vi "Parse-broadcast-data-status.vi"(8 "error in (no error)":errorcluster, 10 "Multiple device identification XML string":string="<LecList>\n  <Lec name='EC_Alpha' ip='192.168.42.30' mac='address' />\n  <Lec name='EC_Beta' ip='192.168.42.31' mac='addressB' />\n</LecList>") -> (0 "error out":errorcluster, 2 "Status information":T1)   [LabVIEW 2013, in "HardwareCharacterization.lvlib" / "HC-SM1000.lvclass"]
uses:
  HC-SM1000.lvclass
  Status-information.ctl
  <vilib>/xml/Load XML String.vi
  <vilib>/xml/Close Reference(Node).vi
  <vilib>/xml/NI_XML.lvlib
  <resource>/objmgr/DOMUserDefRef.rc
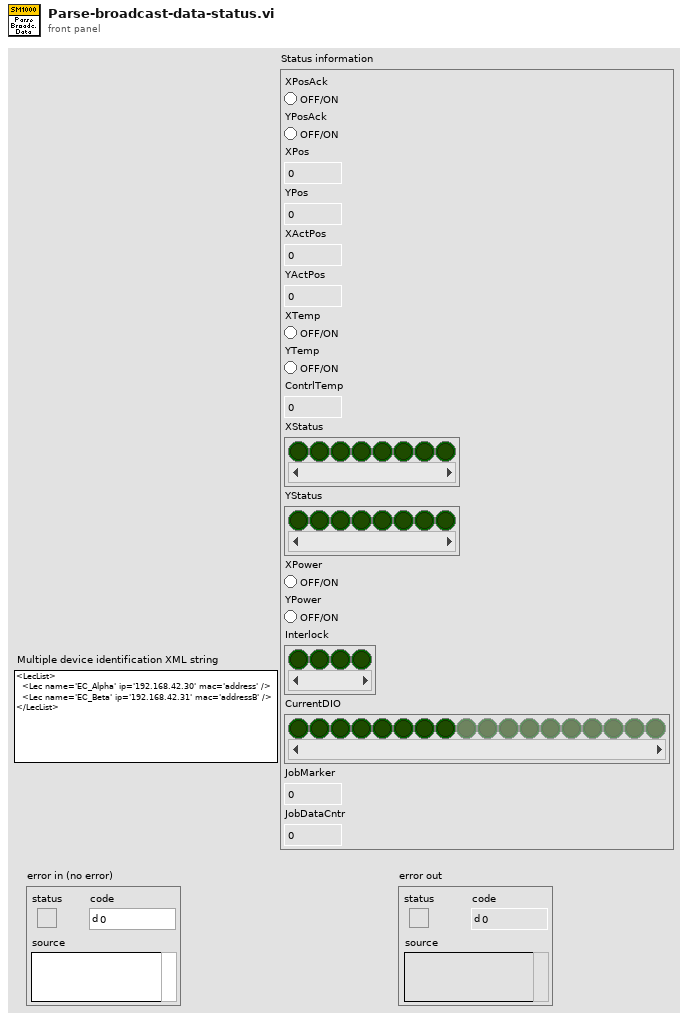
[diagram p1: front panel]
types:
  T1 = typedef "HardwareCharacterization.lvlib/HC-SM1000.lvclass/Status-information.ctl" = cluster{"XPosAck":bool, "YPosAck":bool, "XPos":i16, "YPos":i16, "XActPos":i16, "YActPos":i16, "XTemp":bool, "YTemp":bool, "ContrlTemp":i16, "XStatus":bool[], "YStatus":bool[], "XPower":bool, "YPower":bool, "Interlock":bool[], "CurrentDIO":bool[], "JobMarker":u16, "JobDataCntr":u32}
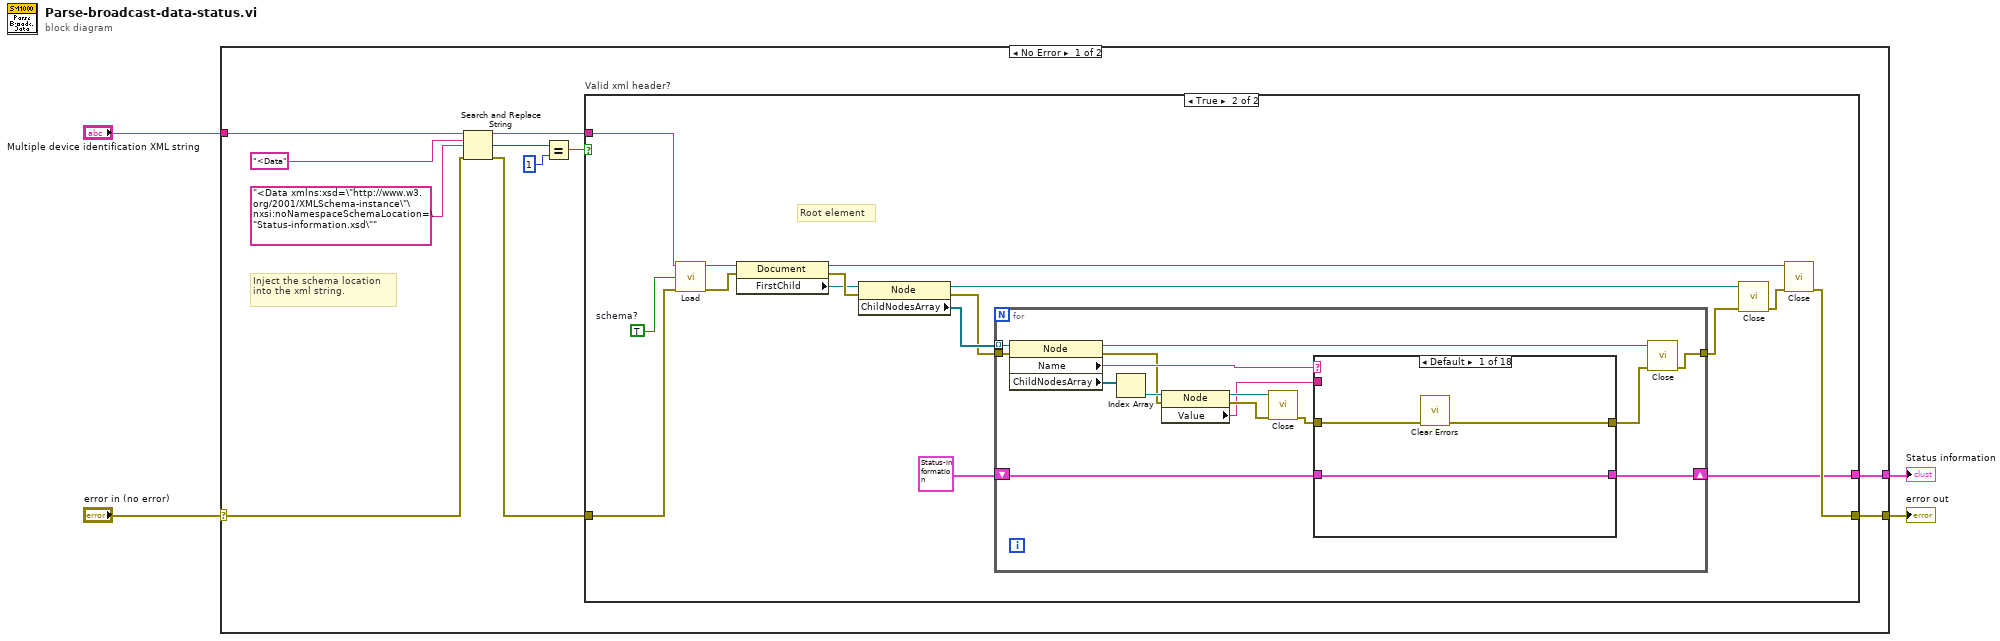
[diagram p0: block diagram]
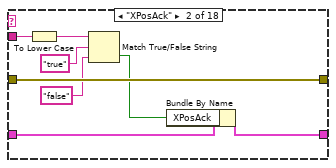
[diagram p3: hidden frame]
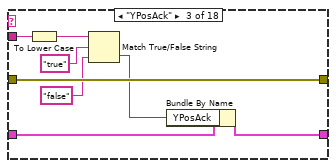
[diagram p4: hidden frame]
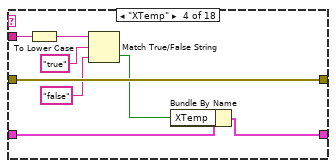
[diagram p5: hidden frame]
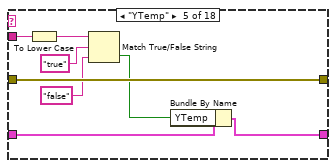
[diagram p6: hidden frame]
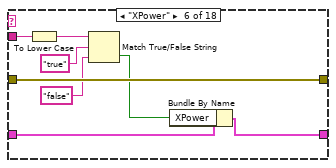
[diagram p7: hidden frame]
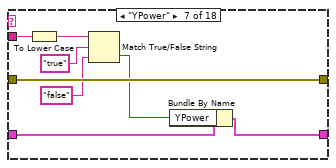
[diagram p8: hidden frame]
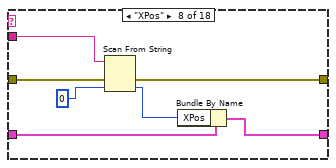
[diagram p9: hidden frame]
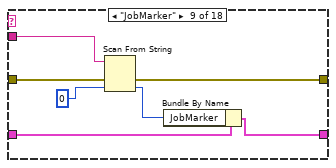
[diagram p10: hidden frame]
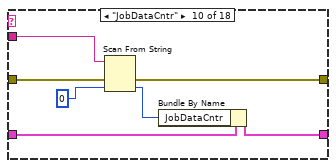
[diagram p11: hidden frame]
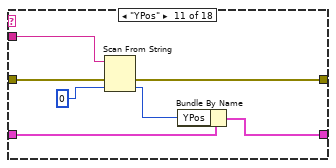
[diagram p12: hidden frame]
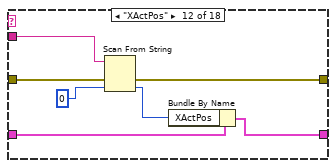
[diagram p13: hidden frame]
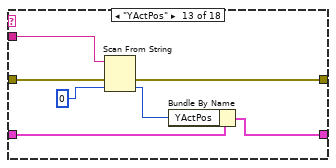
[diagram p14: hidden frame]
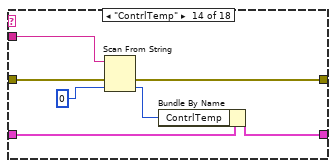
[diagram p15: hidden frame]
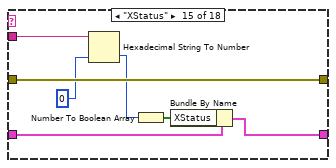
[diagram p16: hidden frame]
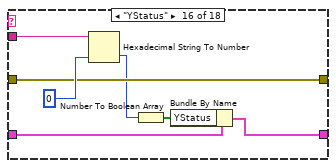
[diagram p17: hidden frame]
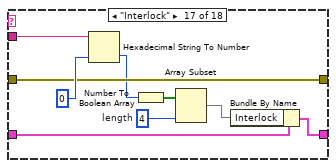
[diagram p18: hidden frame]
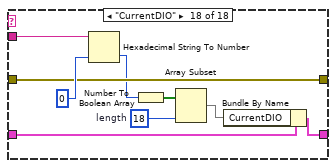
[diagram p19: hidden frame]
diagram:
  n1 = case shown="No Error" "error in (no error)" {
    selector: "error in (no error)" -> [w12 w180]
    tunnel: [w7 w180] -> w3
    tunnel: "Multiple device identification XML string" -> [w15 _]
    tunnel: [w5 _] -> w1
    frame No Error {
      # "Inject the schema location\ninto the xml string."
      n2 = Search and Replace String(input string=w15, search string="<Data", replace string="<Data xmlns:xsd=\"http://www.w3.org/2001/XMLSchema-instance\"\nxsi:noNamespaceSchemaLocation=\"Status-information.xsd\"", error in=w12) -> (result string=w8:string, number of replacements=w11:i32, error out=w6:errorcluster)  [unwired: 4 in, 1 out]
      n3 = Equal?(x=w11, y=1) -> (x = y?=w9:bool)
      n4 = case "Valid xml header?" shown="True" w9 {
        tunnel: w8 -> [_ w19]
        tunnel: [w16 w28] -> w7
        tunnel: w6 -> [w16 w29]
        tunnel: [_ w17] -> w5
        frame False {
        }
        frame True {
          w32 = TRUE  # schema?
          # "Root element"
          n5 = call-poly <vilib>:"Load.vi"("XML string"=w19, "process schema (False)"=w32, "error in (no error)"=w29) -> ("DOM document out"=w31:refnum<k20>, "error out"=w30:errorcluster)  [unwired: 10 in, 1 out]
          n6 = property class="Document"(reference=w31, error in=w30) -> (reference out=w21:refnum<k20>, error out=w23:errorcluster, "FirstChild"=w20:refnum<k20>)
          n7 = property class="Node"(reference=w20, error in=w23) -> (reference out=w22:refnum<k20>, error out=w24:errorcluster, "ChildNodesArray"=w25:refnum<k20>[])
          n8 = for {
            tunnel: w25 -> [w47] mode=indexing
            tunnel: w24 -> [w46]
            tunnel: [w43] -> w27
            shift-right: [w40] -> w17
            shift-left: T1 {"XPosAck"=FALSE, "YPosAck"=FALSE, "XPos"=0, "YPos"=0, "XActPos"=0, "YActPos"=0, "XTemp"=FALSE, "YTemp"=FALSE, "ContrlTemp"=0, "XStatus"=[FALSE, FALSE, FALSE, FALSE, FALSE, FALSE, FALSE, FALSE], "YStatus"=[FALSE, FALSE, FALSE, FALSE, FALSE, FALSE, FALSE, FALSE], "XPower"=FALSE, "YPower"=FALSE, "Interlock"=[FALSE, FALSE, FALSE, FALSE], "CurrentDIO"=[FALSE, FALSE, FALSE, FALSE, FALSE, FALSE, FALSE, FALSE, FALSE, FALSE, FALSE, FALSE, FALSE, FALSE, FALSE, FALSE, FALSE, FALSE], "JobMarker"=0, "JobDataCntr"=0} ("Status information") -> [w41]
            n9 = property class="Node"(reference=w47, error in=w46) -> (reference out=w45:refnum<k20>, error out=w37:errorcluster, "Name"=w42:string, "ChildNodesArray"=w39:refnum<k20>[])
            n10 = Index Array(array=w39) -> (element=w38:refnum<k20>)  [unwired: 1 in]
            n11 = property class="Node"(reference=w38, error in=w37) -> (reference out=w34:refnum<k20>, error out=w36:errorcluster, "Value"=w33:string)
            n12 = call-poly <vilib>:"Close.vi"("error in (no error)"=w36, "node"=w34) -> ("error out"=w35:errorcluster)  [unwired: 7 in]
            n13 = case shown="Default" w42 {
              tunnel: w35 -> [w50 w55 w63 w71 w79 w87 w95 w103 w110 w117 w124 w131 w138 w145 w150 w156 w163 w172]
              tunnel: [w48 w55 w63 w71 w79 w87 w95 w99 w106 w113 w120 w127 w134 w141 w150 w156 w163 w172] -> w44
              tunnel: w41 -> [w49 w58 w66 w74 w82 w90 w98 w105 w112 w119 w126 w133 w140 w147 w154 w161 w170 w179]
              tunnel: w33 -> [_ w56 w64 w72 w80 w88 w96 w102 w109 w116 w123 w130 w137 w144 w152 w157 w164 w173]
              tunnel: [w49 w57 w65 w73 w81 w89 w97 w104 w111 w118 w125 w132 w139 w146 w153 w160 w169 w178] -> w40
              frame Default {
                n14 = call <vilib>:"Clear Errors.vi"("error in (no error)"=w50) -> ("error out"=w48:errorcluster)  [unwired: 6 in]
              }
              frame "XPosAck" {
                n15 = To Lower Case(string=w56) -> (all lower case string=w54:string)
                n16 = Match True/False String(2:"false", 3:"true", 4:w54) -> (0:w51:bool)  [unwired: 1 out]
                n17 = Bundle By Name(cluster=w58, "XPosAck"=w51) -> (w57:T1)
              }
              frame "YPosAck" {
                n18 = To Lower Case(string=w64) -> (all lower case string=w62:string)
                n19 = Match True/False String(2:"false", 3:"true", 4:w62) -> (0:w59:bool)  [unwired: 1 out]
                n20 = Bundle By Name(cluster=w66, "YPosAck"=w59) -> (w65:T1)
              }
              frame "XTemp" {
                n21 = To Lower Case(string=w72) -> (all lower case string=w70:string)
                n22 = Match True/False String(2:"false", 3:"true", 4:w70) -> (0:w67:bool)  [unwired: 1 out]
                n23 = Bundle By Name(cluster=w74, "XTemp"=w67) -> (w73:T1)
              }
              frame "YTemp" {
                n24 = To Lower Case(string=w80) -> (all lower case string=w78:string)
                n25 = Match True/False String(2:"false", 3:"true", 4:w78) -> (0:w75:bool)  [unwired: 1 out]
                n26 = Bundle By Name(cluster=w82, "YTemp"=w75) -> (w81:T1)
              }
              frame "XPower" {
                n27 = To Lower Case(string=w88) -> (all lower case string=w86:string)
                n28 = Match True/False String(2:"false", 3:"true", 4:w86) -> (0:w83:bool)  [unwired: 1 out]
                n29 = Bundle By Name(cluster=w90, "XPower"=w83) -> (w89:T1)
              }
              frame "YPower" {
                n30 = To Lower Case(string=w96) -> (all lower case string=w94:string)
                n31 = Match True/False String(2:"false", 3:"true", 4:w94) -> (0:w91:bool)  [unwired: 1 out]
                n32 = Bundle By Name(cluster=w98, "YPower"=w91) -> (w97:T1)
              }
              frame "XPos" {
                n33 = Scan From String(input string=w102, error in=w103, default 1=i16 0) -> (error out=w99:errorcluster, output 1=w100:i16)  [unwired: 2 in, 2 out]
                n34 = Bundle By Name(cluster=w105, "XPos"=w100) -> (w104:T1)
              }
              frame "JobMarker" {
                n35 = Scan From String(input string=w109, error in=w110, default 1=u16 0) -> (error out=w106:errorcluster, output 1=w107:u16)  [unwired: 2 in, 2 out]
                n36 = Bundle By Name(cluster=w112, "JobMarker"=w107) -> (w111:T1)
              }
              frame "JobDataCntr" {
                n37 = Scan From String(input string=w116, error in=w117, default 1=u32 0) -> (error out=w113:errorcluster, output 1=w114:u32)  [unwired: 2 in, 2 out]
                n38 = Bundle By Name(cluster=w119, "JobDataCntr"=w114) -> (w118:T1)
              }
              frame "YPos" {
                n39 = Scan From String(input string=w123, error in=w124, default 1=i16 0) -> (error out=w120:errorcluster, output 1=w121:i16)  [unwired: 2 in, 2 out]
                n40 = Bundle By Name(cluster=w126, "YPos"=w121) -> (w125:T1)
              }
              frame "XActPos" {
                n41 = Scan From String(input string=w130, error in=w131, default 1=i16 0) -> (error out=w127:errorcluster, output 1=w128:i16)  [unwired: 2 in, 2 out]
                n42 = Bundle By Name(cluster=w133, "XActPos"=w128) -> (w132:T1)
              }
              frame "YActPos" {
                n43 = Scan From String(input string=w137, error in=w138, default 1=i16 0) -> (error out=w134:errorcluster, output 1=w135:i16)  [unwired: 2 in, 2 out]
                n44 = Bundle By Name(cluster=w140, "YActPos"=w135) -> (w139:T1)
              }
              frame "ContrlTemp" {
                n45 = Scan From String(input string=w144, error in=w145, default 1=i16 0) -> (error out=w141:errorcluster, output 1=w142:i16)  [unwired: 2 in, 2 out]
                n46 = Bundle By Name(cluster=w147, "ContrlTemp"=w142) -> (w146:T1)
              }
              frame "XStatus" {
                n47 = Hexadecimal String To Number(string=w152, default (0uL)=u8 0) -> (number=w148:u8)  [unwired: 1 in, 1 out]
                n48 = Number To Boolean Array(number=w148) -> (Boolean array=w151:bool[])
                n49 = Bundle By Name(cluster=w154, "XStatus"=w151) -> (w153:T1)
              }
              frame "YStatus" {
                n50 = Hexadecimal String To Number(string=w157, default (0uL)=u8 0) -> (number=w155:u8)  [unwired: 1 in, 1 out]
                n51 = Number To Boolean Array(number=w155) -> (Boolean array=w159:bool[])
                n52 = Bundle By Name(cluster=w161, "YStatus"=w159) -> (w160:T1)
              }
              frame "Interlock" {
                w166 = 4  # length
                n53 = Hexadecimal String To Number(string=w164, default (0uL)=u32 0) -> (number=w162:u32)  [unwired: 1 in, 1 out]
                n54 = Number To Boolean Array(number=w162) -> (Boolean array=w167:bool[])
                n55 = Array Subset(array=w167, length=w166) -> (w168:bool[])  [unwired: 1 in]
                n56 = Bundle By Name(cluster=w170, "Interlock"=w168) -> (w169:T1)
              }
              frame "CurrentDIO" {
                w175 = 18  # length
                n57 = Hexadecimal String To Number(string=w173, default (0uL)=u32 0) -> (number=w171:u32)  [unwired: 1 in, 1 out]
                n58 = Number To Boolean Array(number=w171) -> (Boolean array=w176:bool[])
                n59 = Array Subset(array=w176, length=w175) -> (w177:bool[])  [unwired: 1 in]
                n60 = Bundle By Name(cluster=w179, "CurrentDIO"=w177) -> (w178:T1)
              }
            }
            n61 = call-poly <vilib>:"Close.vi"("error in (no error)"=w44, "node"=w45) -> ("error out"=w43:errorcluster)  [unwired: 7 in]
          }
          n62 = call-poly <vilib>:"Close.vi"("error in (no error)"=w27, "node"=w22) -> ("error out"=w26:errorcluster)  [unwired: 7 in]
          n63 = call-poly <vilib>:"Close.vi"("error in (no error)"=w26, "node"=w21) -> ("error out"=w28:errorcluster)  [unwired: 7 in]
        }
      }
    }
    frame Error {
    }
  }
  "error out" <- w3
  "Status information" <- w1
